vi "Convert IE times to brpm.vi"(8 "loop rate":u16=5, 10 "expcounts":u16, 11 "inspcounts":u16) -> (2 "I:E Ratio":T1=6 max=7 step=1 scale=0.0..7.0, 3 "Brpm":sgl=6.0 format="%#_2g")   [LabVIEW 2016]
uses:
  Controls/IE Ratio knob.ctl
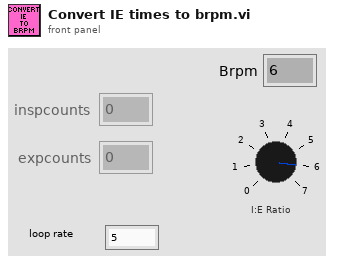
[diagram p1: front panel]
types:
  T1 = typedef "IE Ratio knob.ctl" = u8
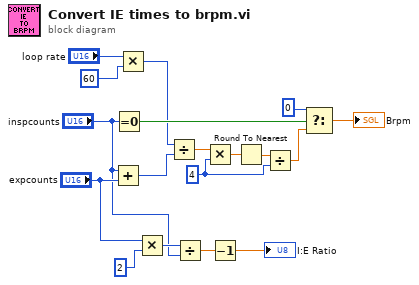
[diagram p0: block diagram]
diagram:
  w4 = 4
  n1 = Add(x="inspcounts", y="expcounts") -> (x+y=w9:u16)
  n2 = Equal To 0?(x="inspcounts") -> (x = 0?=w18:bool)
  n3 = Multiply(x="loop rate", y=u16 60) -> (x*y=w1:u16)
  n4 = Multiply(x="expcounts", y=u16 2) -> (x*y=w14:u16)
  n5 = Divide(x=w1, y=w9) -> (x/y=w8:dbl)
  n6 = Divide(x=w14, y="inspcounts") -> (x/y=w11:dbl)
  n7 = Multiply(x=w8, y=w4) -> (x*y=w7:dbl)
  n8 = Decrement(x=w11) -> (x-1=→"I:E Ratio":dbl)
  n9 = Round To Nearest(number=w7) -> (nearest integer value=w5:dbl)
  n10 = Divide(x=w5, y=w4) -> (x/y=w6:dbl)
  n11 = Select(t=0, s=w18, f=w6) -> (s? t:f=→"Brpm":dbl)
